vi "raport_for_operator.vi"(9 "adres":string, 10 "max":string, 11 "min":string) -> ()   [LabVIEW 2023]
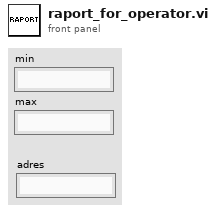
[diagram p1: front panel]
types:
  T1 = enum16{"open", "replace", "create", "open or create", "replace or create", "replace or create with confirmation"}
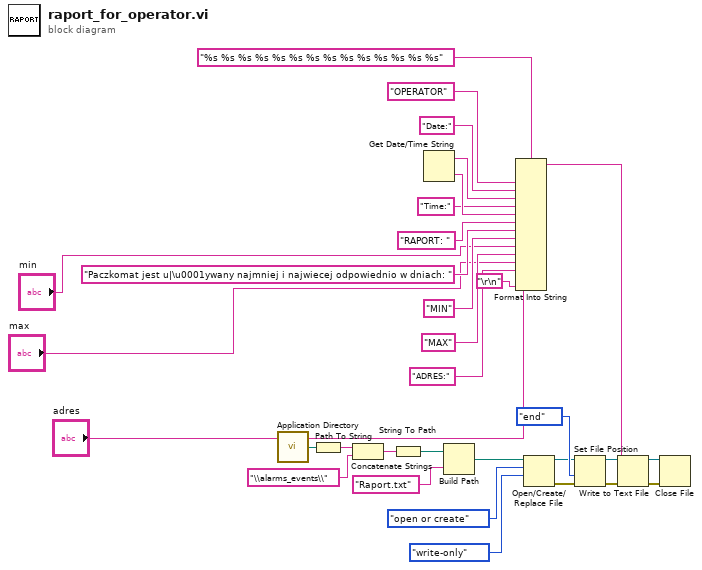
[diagram p0: block diagram]
diagram:
  n1 = call <vilib>:"Application Directory.vi"() -> ("Application Directory"=w26:path)
  n2 = Path To String(path=w26) -> (string=w27:string)
  n3 = Concatenate Strings(w27, "\\alarms_events\\") -> (w29:string)
  n4 = String To Path(string=w29) -> (path=w30:path)
  n5 = Get Date/Time String() -> (date string=w19:string, time string=w21:string)  [unwired: 3 in]
  n6 = Build Path(base path=w30, name or relative path="Raport.txt") -> (appended path=w31:path)
  n7 = Format Into String(format string="%s %s %s %s %s %s %s %s %s %s %s %s %s %s", "OPERATOR" ("name_user_option"), "Date:" ("format string"), w19, "Time:" ("format string"), w21, "RAPORT: " ("format string"), "Paczkomat jest u|\u0001ywany najmniej i najwiecej odpowiednio w dniach: " ("text_raport"), "MIN" ("input 8"), "min", "MAX" ("input 10"), "max", "ADRES:" ("input 9"), "adres", "\r\n") -> (resulting string=w24:string)  [unwired: 2 in, 1 out]
  n8 = Open/Create/Replace File(file path (use dialog)=w31, operation (0:open)=T1."open or create", access (0:read/write)=enum16{"read/write", "read-only", "write-only"}."write-only") -> (refnum out=w10:refnum<file>, error out=w9:errorcluster)  [unwired: 3 in, 1 out]
  n9 = Set File Position(refnum=w10, from (0:start)=enum16{"start", "end", "current"}."end", error in=w9) -> (refnum out=w13:refnum<file>, error out=w14:errorcluster)  [unwired: 1 in]
  n10 = Write to Text File(file (use dialog)=w13, text=w24, error in=w14) -> (refnum out=w12:refnum<file>, error out=w11:errorcluster)  [unwired: 1 in, 1 out]
  n11 = Close File(refnum=w12, error in=w11) -> ()  [unwired: 2 out]
